vi "Set Voltage type.vi"(8 "error in (no error)":errorcluster caption="entrée d'erreur (pas d'erreur)", 10 "Voltage Type":enum16{"AC", "DC"}(ring), 11 "Class Multimeter (Default) en entrée":refnum<class "Class Multimeter (Default).lvclass">) -> (0 "error out":errorcluster caption="sortie d'erreur", 3 "Class Multimeter (Default) en sortie":refnum<class "Class Multimeter (Default).lvclass">)   [LabVIEW 2020, in "Library Instrument & Equipement.lvlib" / "Library Multimeter.lvlib" / "Class Multimeter (Default).lvclass"]
uses:
  Class Multimeter (Default).lvclass
  Class Multimeter (Default).lvclass/Class Multimeter (Default).ctl
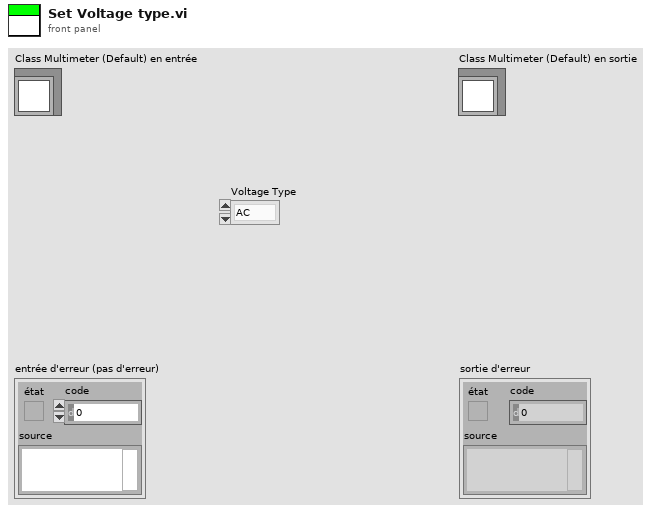
[diagram p1: front panel]
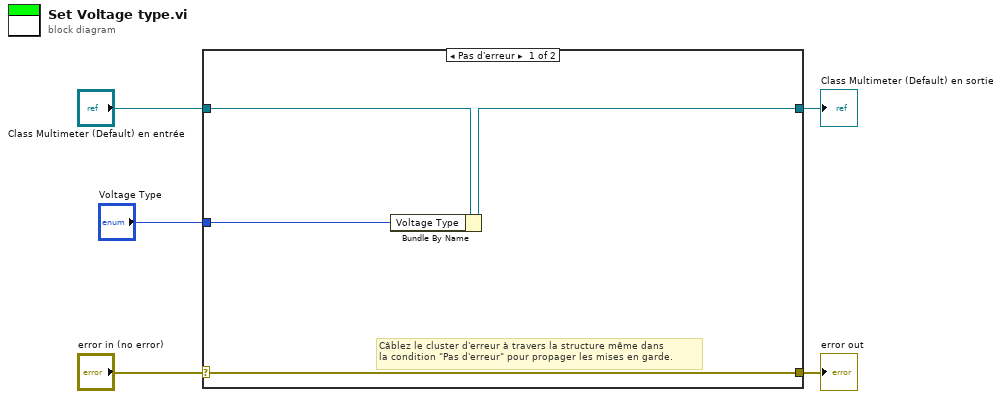
[diagram p0: block diagram]
diagram:
  n1 = case shown="Pas d'erreur" "error in (no error)" {
    selector: "error in (no error)" -> [w9 w11]
    tunnel: [w9 w11] -> w4
    tunnel: [w7 w10] -> w2
    tunnel: "Class Multimeter (Default) en entrée" -> [w8 w10]
    tunnel: "Voltage Type" -> [w6 _]
    frame No Error {
      # "Câblez le cluster d'erreur à travers la structure même dans\nla condition \"Pas d'erreur\" pour propager les mises en garde."
      n2 = Bundle By Name(cluster=w8, "Voltage Type"=w6) -> (w7:refnum<class "Class Multimeter (Default).lvclass">)
    }
    frame Error {
    }
  }
  "error out" <- w4
  "Class Multimeter (Default) en sortie" <- w2
